vi "3D Scanner - Servo - MANUAL.vi"() -> ()   [LabVIEW 2012]
uses:
  <vilib>/Instr/_visa.llb/VISA Configure Serial Port (Instr).vi
panel:
  in  "Select COM Port":refnum<visa-resource-name>="COM4"
  in  "Left/Right":u8(slide) scale=0.0..254.0
  in  "Up/Down":u8(slide) scale=0.0..254.0
  in  "Platform":u8(slide) scale=0.0..254.0
  in  "stop":bool
  # "3D Scanner servo Controller"
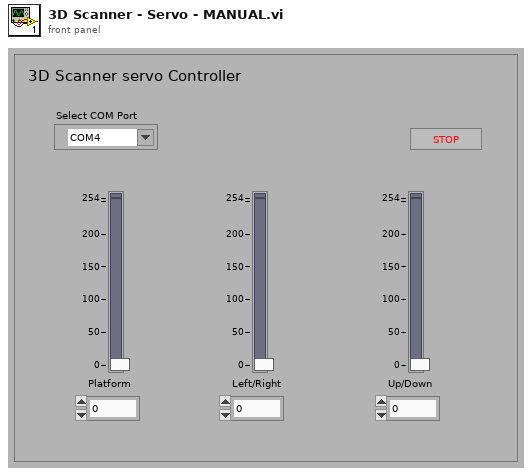
[diagram p1: front panel]
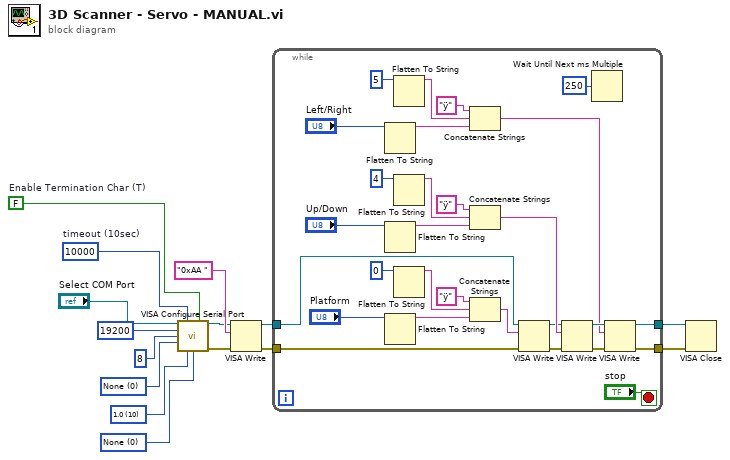
[diagram p0: block diagram]
diagram:
  w5 = u16 0 items=["None"=0, "XON/XOFF"=1, "RTS/CTS"=2, "DTR/DSR"=4] ("flow control")
  w6 = u16 10 items=["1.0"=10, "1.5"=15, "2.0"=20] ("stop bits")
  w7 = u16 0 items=["None", "Odd", "Even", "Mark", "Space"] ("parity")
  w11 = FALSE  # Enable Termination Char (T)
  w12 = u32 10000  # timeout (10sec)
  n1 = call-poly "VISA Configure Serial Port"("VISA resource name"="Select COM Port", "timeout (10sec)"=w12, "Enable Termination\nChar (T)"=w11, "baud rate (9600)"=u32 19200 ("baud rate"), "data bits (8)"=u16 8 ("data bits"), "parity (0:none)"=w7, "stop bits (10: 1 bit)"=w6, "flow control (0:none)"=w5) -> ("VISA resource name out"=w3:refnum<visa-resource-name>, "error out"=w4:errorcluster)  [unwired: 1 in, 5 out]
  n2 = VISA Write(VISA resource name=w3, write buffer="0xAA ", error in (no error)=w4) -> (VISA resource name out=w14:refnum<visa-resource-name>, error out=w13:errorcluster)  [unwired: 1 out]
  n3 = while {
    tunnel: w14 -> [w39]
    tunnel: w13 -> [w38]
    tunnel: [w21] -> w2
    tunnel: [w20] -> w1
    stop <- "stop" stop-if-true
    n4 = Flatten To String(anything="Left/Right") -> (data string=w26:string)  [unwired: 1 in, 4 out]
    n5 = Flatten To String(anything="Up/Down") -> (data string=w31:string)  [unwired: 1 in, 4 out]
    n6 = Flatten To String(anything="Platform") -> (data string=w41:string)  [unwired: 1 in, 4 out]
    n7 = Flatten To String(anything=5) -> (data string=w27:string)  [unwired: 1 in, 4 out]
    n8 = Flatten To String(anything=4) -> (data string=w32:string)  [unwired: 1 in, 4 out]
    n9 = Flatten To String(anything=0) -> (data string=w42:string)  [unwired: 1 in, 4 out]
    n10 = Concatenate Strings("ÿ", w27, w26) -> (w16:string)
    n11 = Concatenate Strings("ÿ", w32, w31) -> (w19:string)
    n12 = Concatenate Strings("ÿ", w42, w41) -> (w40:string)
    n13 = VISA Write(VISA resource name=w39, write buffer=w40, error in (no error)=w38) -> (VISA resource name out=w18:refnum<visa-resource-name>, error out=w23:errorcluster)  [unwired: 1 out]
    n14 = VISA Write(VISA resource name=w18, write buffer=w19, error in (no error)=w23) -> (VISA resource name out=w17:refnum<visa-resource-name>, error out=w22:errorcluster)  [unwired: 1 out]
    n15 = Wait Until Next ms Multiple(millisecond multiple=250) -> ()  [unwired: 1 out]
    n16 = VISA Write(VISA resource name=w17, write buffer=w16, error in (no error)=w22) -> (VISA resource name out=w20:refnum<visa-resource-name>, error out=w21:errorcluster)  [unwired: 1 out]
  }
  n17 = VISA Close(VISA resource name=w1, error in (no error)=w2) -> ()  [unwired: 1 out]
